vi "OxITC503 _Query_ Examine ITC503 Status.vi"(0 "VISA session":refnum<visa-resource-name>="GPIB::2", 1 "error in":errorcluster) -> (2 "VISA session":refnum<visa-resource-name>, 3 "ITC Status":T1, 4 "error out (no error)":errorcluster, 5 "Initialising Needle Valve":bool caption="Initialising Needle Valve?")   [LabVIEW 2013]
doc: "Reads the current ITC503 STATUS. It requires no parameters."
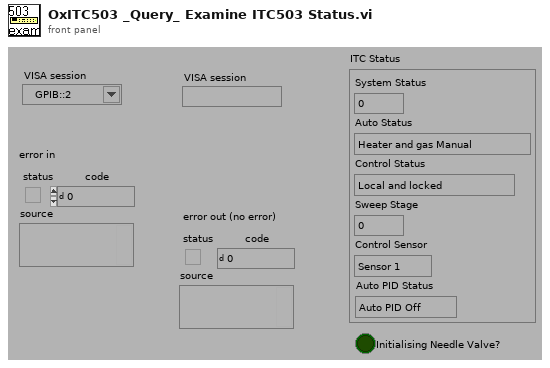
[diagram p1: front panel]
types:
  T1 = cluster{"System Status":i32, "Auto Status":enum16{"Heater and gas Manual", "Heater Auto, Gas Manual", "Heater Manual, Gas Auto", "Heater and Gas Auto"}, "Control Status":enum16{"Local and locked", "Remote and Locked", "Local and unlocked", "Remote and Unlocked"}, "Sweep Stage":i32, "Control Sensor":enum16{"Sensor 1", "Sensor 2", "Sensor 3"}, "Auto PID Status":enum16{"Auto PID Off", "Auto PID On"}}
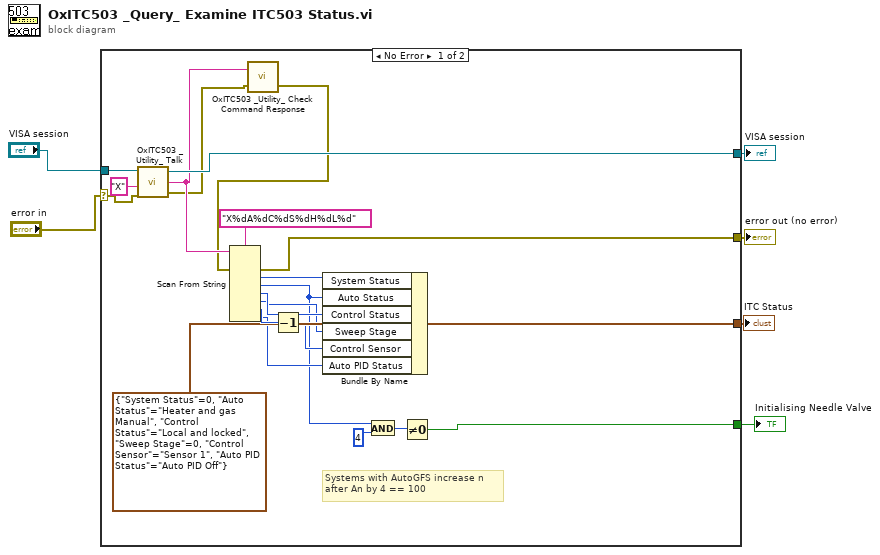
[diagram p0: block diagram]
diagram:
  n1 = case shown="No Error" "error in" {
    selector: "error in" -> [w11 w28]
    tunnel: [w27 w29] -> w6
    tunnel: "VISA session" -> [w26 w29]
    tunnel: [w19 _] -> w4
    tunnel: [w17 w28] -> w3
    tunnel: [w7 _] -> w1
    frame No Error {
      # "Systems with AutoGFS increase n \nafter An by 4 == 100"
      n2 = call "OxITC503 _Utility_ Talk.vi"("VISA session"=w26, "Command"="X", "error in (no error)"=w11) -> ("VISA session"=w27:refnum<visa-resource-name>, "read buffer"=w22:string, "error out (no error)"=w21:errorcluster)  [unwired: 2 in]
      n3 = call "OxITC503 _Utility_ Check Command Response.vi"("error in"=w21, "read buffer"=w22) -> ("error out (no error)"=w20:errorcluster)  [unwired: 1 out]
      n4 = Scan From String(format string="X%dA%dC%dS%dH%dL%d" ("Format String"), input string=w22, error in=w20) -> (error out=w17:errorcluster, output 1=w16:i32, output 2=w8:i32, output 3=w15:i32, output 4=w14:i32, output 5=w23:i32, output 6=w12:i32)  [unwired: 7 in, 2 out]
      n5 = Decrement(x=w23) -> (x-1=w13:i32)
      n6 = Bundle By Name(cluster=T1 {"System Status"=0, "Auto Status"=enum."Heater and gas Manual", "Control Status"=enum."Local and locked", "Sweep Stage"=0, "Control Sensor"=enum."Sensor 1", "Auto PID Status"=enum."Auto PID Off"} ("ITC Status 2"), "System Status"=w16, "Auto Status"=w8, "Control Status"=w15, "Sweep Stage"=w14, "Control Sensor"=w13, "Auto PID Status"=w12) -> (w19:T1)
      n7 = And(x=w8, y=4) -> (x .and. y?=w10:i32)
      n8 = Not Equal To 0?(x=w10) -> (x != 0?=w7:bool)
    }
    frame Error {
    }
  }
  "error out (no error)" <- w3
  "VISA session" <- w6
  "ITC Status" <- w4
  "Initialising Needle Valve" <- w1
